vi "数据补传对话框.vi"() -> (2 "输出":bool=TRUE, 3 "时间OUT":timestamp)   [LabVIEW 2016, in "中水三立SQL数据传输.lvlib"]
panel:
  in  "取消":bool
  in  "确定":bool
  in  "起始时间":timestamp
  # "数据补传时间选择"
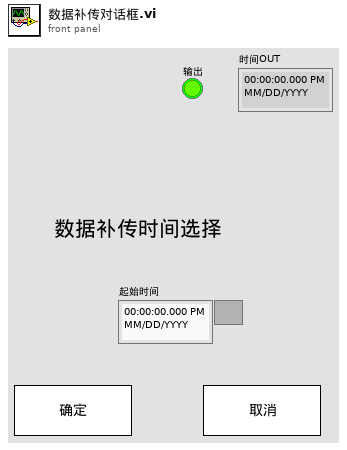
[diagram p1: front panel]
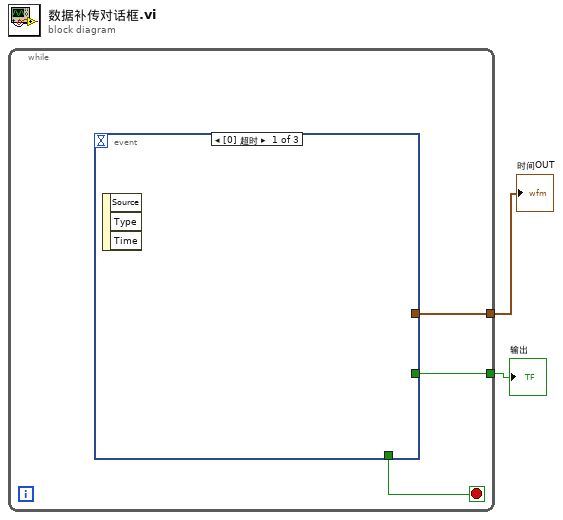
[diagram p0: block diagram]
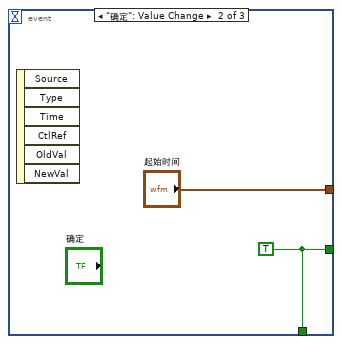
[diagram p2: hidden frame]
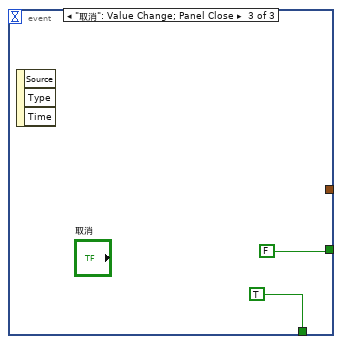
[diagram p3: hidden frame]
diagram:
  n1 = while {
    tunnel: [w5] -> w2
    tunnel: [w4] -> w1
    stop <- w3 stop-if-true
    n2 = event shown="[0] 超时" {
      selector: _ -> [_ _ _]
      dyn-events: _ -> [_ _ _]
      timeout: _ -> [_ _ _]
      tunnel: [_ w6 FALSE] -> w5
      tunnel: [_ "起始时间" _] -> w4
      tunnel: [_ w6 TRUE] -> w3
      event Timeout {
        n3 = event-data() -> ()  [unwired: 1 in, 3 out]
      }
      event "确定": Value Change {
        w6 = TRUE
        n4 = event-data() -> ()  [unwired: 1 in, 6 out]
      }
      event "取消": Value Change; Panel Close {
        n5 = event-data() -> ()  [unwired: 1 in, 3 out]
      }
    }
  }
  "输出" <- w2
  "时间OUT" <- w1
